vi "Compute.vi"(8 "error in (no error)":errorcluster, 9 "Data Channels":T1, 10 "x-var":dbl, 11 "Norm in":refnum<class "Norm.lvclass">) -> (0 "error out":errorcluster, 1 "Add'l Data Channels":T1, 3 "Norm out":refnum<class "Norm.lvclass">)   [LabVIEW 2009, in "Norm.lvclass"]
doc: "Given a data channel and an x-coordinate, compute and return one or more new data channels."
uses:
  Norm.lvclass
  Instruments/Utility Classes/Readable/Data Channels.ctl
  Instruments/Utility Classes/Readable/Data Channel.ctl
  Instruments/Utility Classes/Readable/Data Point.ctl
  Instruments/Utility Classes/Readable/Readable.lvclass
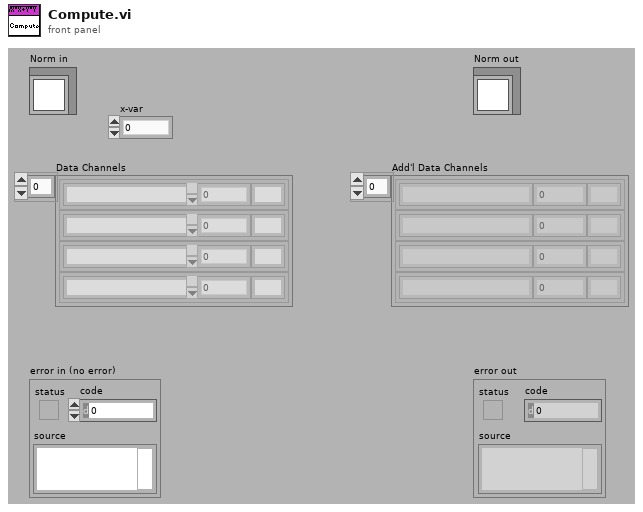
[diagram p1: front panel]
types:
  T1 = typedef "Readable.lvclass/Data Channels.ctl" = T2[]
  T2 = typedef "Readable.lvclass/Data Channel.ctl" = cluster{"Name":string, "Data Point":T3, "Unit":string}
  T3 = typedef "Readable.lvclass/Data Point.ctl" = dbl
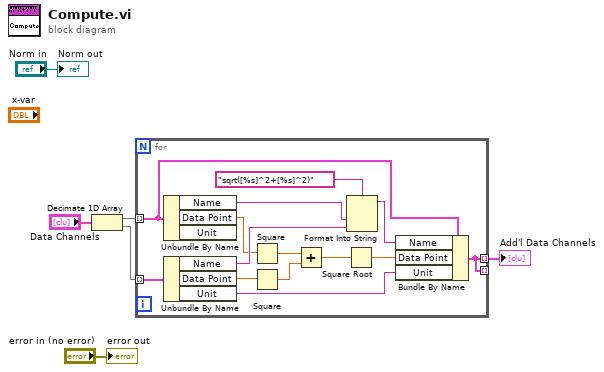
[diagram p0: block diagram]
diagram:
  n1 = Decimate 1D Array("Data Channels") -> (w6:T2[], w5:T2[])
  n2 = for {
    tunnel: w6 -> [w16] mode=indexing
    tunnel: w5 -> [w20] mode=indexing
    tunnel: [w10] -> _ mode=indexing
    tunnel: [w10] -> w3 mode=indexing
    n3 = Unbundle By Name(w16) -> ("Name"=w18:string, "Data Point"=w13:T3)  [unwired: 1 out]
    n4 = Unbundle By Name(w20) -> ("Name"=w17:string, "Data Point"=w12:T3, "Unit"=w15:string)
    n5 = Square(x=w13) -> (x^2=w9:T3)
    n6 = Square(x=w12) -> (x^2=w8:T3)
    n7 = Add(x=w9, y=w8) -> (x+y=w11:T3)
    n8 = Square Root(x=w11) -> (sqrt(x)=w7:T3)
    n9 = Format Into String(format string="sqrt([%s]^2+[%s]^2)", w18, w17) -> (resulting string=w14:string)  [unwired: 2 in, 1 out]
    n10 = Bundle By Name(cluster=w16, "Name"=w14, "Data Point"=w7, "Unit"=w15) -> (w10:T2)
  }
  "Add'l Data Channels" <- w3
  "error out" <- "error in (no error)"
  "Norm out" <- "Norm in"
